vi "Write command to PG.vi"(8 "error in (no error)":errorcluster, 10 "Write Buffer":string, 11 "VISA resource name":refnum<visa-resource-name>) -> (0 "error out":errorcluster, 2 "Read Buffer":string, 3 "VISA resource name out":refnum<visa-resource-name>)   [LabVIEW 2018]
uses:
  <vilib>/Utility/error.llb/DialogType.ctl
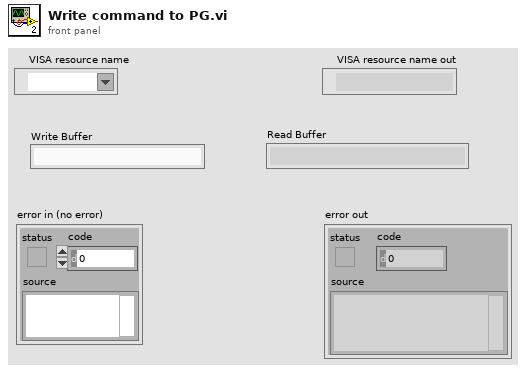
[diagram p1: front panel]
types:
  T1 = typedef "DialogType.ctl" = u16
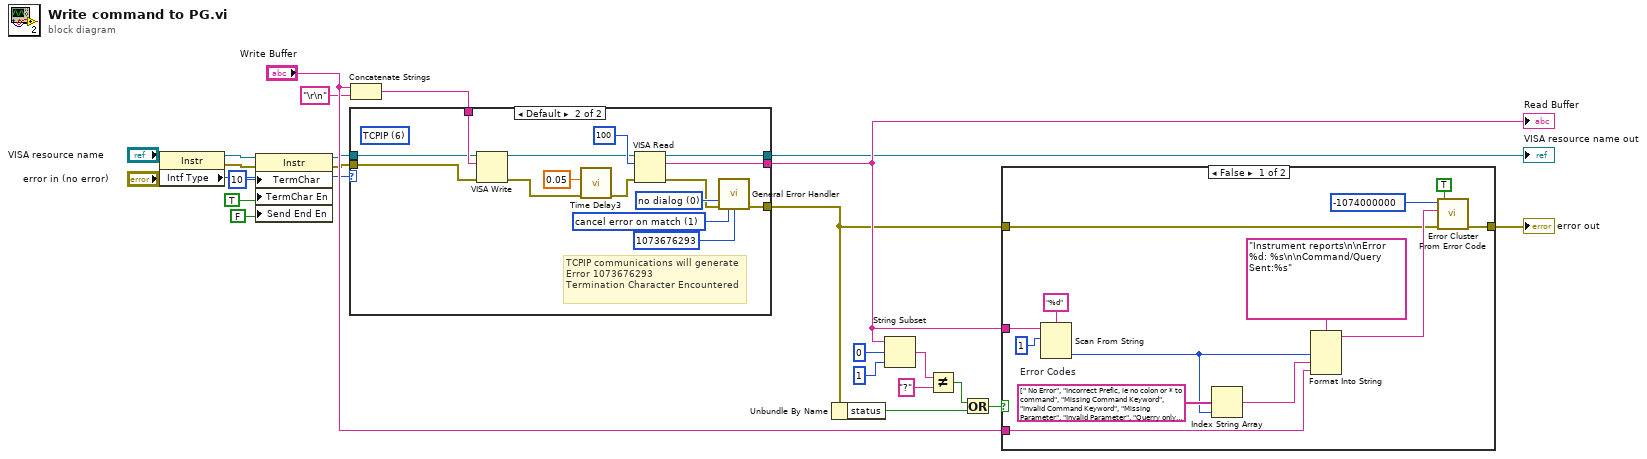
[diagram p0: block diagram]
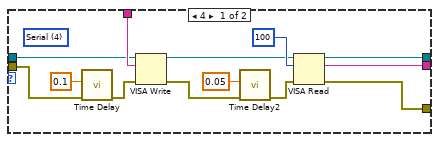
[diagram p2: hidden frame]
diagram:
  n1 = property class="Instr"(reference="VISA resource name", error in="error in (no error)") -> (reference out=w6:refnum<visa-resource-name>, error out=w7:errorcluster, "Intf Type"=w9:u16)
  n2 = property class="Instr"(reference=w6, error in=w7, "TermChar"=u8 10 ("Message Based Settings:Termination Character"), "TermChar En"=TRUE ("Message Based Settings:Termination Character Enable"), "Send End En"=FALSE ("Message Based Settings:Send End Enable")) -> (reference out=w5:refnum<visa-resource-name>, error out=w4:errorcluster)
  n3 = Concatenate Strings("Write Buffer", "\r\n" ("string")) -> (w24:string)
  n4 = case shown="Default" w9 {
    tunnel: w24 -> [w37 w52]
    tunnel: [w35 w50] -> w19
    tunnel: [w34 w49] -> w14
    tunnel: [w33 w38] -> w8
    tunnel: w5 -> [w29 w46]
    tunnel: w4 -> [w28 w43]
    frame 4 {
      (unwired) u16 4 items=["GPIB"=1, "VXI"=2, "GPIB-VXI"=3, "Serial"=4, "PXI"=5, "TCPIP"=6, "USB"=7, "FireWire"=9] ("Interface Information:Interface Type")
      n5 = call "Time Delay"("error in (no error)"=w28, "Delay Time (s)"=0.1) -> ("error out"=w30:errorcluster)  [unwired: 9 out]
      n6 = VISA Write(VISA resource name=w29, write buffer=w37, error in (no error)=w30) -> (VISA resource name out=w27:refnum<visa-resource-name>, error out=w31:errorcluster)  [unwired: 1 out]
      n7 = call "Time Delay2"("error in (no error)"=w31, "Delay Time (s)"=0.05) -> ("error out"=w32:errorcluster)  [unwired: 9 out]
      n8 = VISA Read(VISA resource name=w27, byte count=u32 100, error in (no error)=w32) -> (VISA resource name out=w34:refnum<visa-resource-name>, read buffer=w35:string, error out=w33:errorcluster)  [unwired: 1 out]
    }
    frame Default {
      w42 = T1 0 items=["no dialog", "OK message", "continue or stop message", "OK message + warnings", "continue/stop + warnings"] ("type of dialog (OK msg:1)")
      (unwired) u16 6 items=["GPIB"=1, "VXI"=2, "GPIB-VXI"=3, "Serial"=4, "PXI"=5, "TCPIP"=6, "USB"=7, "FireWire"=9] ("Interface Information:Interface Type")
      w40 = 1 items=["no exception", "cancel error on match", "set error on match"] ("[exception action] (none:0)")
      # "TCPIP communications will generate\nError 1073676293\nTermination Character Encountered"
      n9 = VISA Write(VISA resource name=w46, write buffer=w52, error in (no error)=w43) -> (VISA resource name out=w45:refnum<visa-resource-name>, error out=w47:errorcluster)  [unwired: 1 out]
      n10 = call "Time Delay3"("error in (no error)"=w47, "Delay Time (s)"=0.05) -> ("error out"=w48:errorcluster)  [unwired: 9 out]
      n11 = VISA Read(VISA resource name=w45, byte count=u32 100, error in (no error)=w48) -> (VISA resource name out=w49:refnum<visa-resource-name>, read buffer=w50:string, error out=w39:errorcluster)  [unwired: 1 out]
      n12 = call <vilib>:"General Error Handler.vi"("type of dialog (OK msg:1)"=w42, "error in (no error)"=w39, "[exception action] (none:0)"=w40, "[exception code]"=1073676293) -> ("error out"=w38:errorcluster)  [unwired: 2 in, 9 out]
    }
  }
  "Read Buffer" <- w19
  "VISA resource name out" <- w14
  n13 = Unbundle By Name(w8) -> ("status"=w15:bool)
  n14 = String Subset(string=w19, offset (0)=0, length (rest)=1 ("length (rest)")) -> (substring=w16:string)
  n15 = Not Equal?(x=w16, y="?" ("x")) -> (x != y?=w18:bool)
  n16 = Or(x=w18, y=w15) -> (x .or. y?=w23:bool)
  n17 = case shown="False" w23 {
    tunnel: w19 -> [w64 _]
    tunnel: [w55 w66] -> w22
    tunnel: w8 -> [w53 w66]
    tunnel: "Write Buffer" -> [w59 _]
    frame False {
      w62 = string[] [" No Error", "Incorrect Prefic, ie no colon or * to command", "Missing Command Keyword", "Invalid Command Keyword", "Missing Parameter", "Invalid Parameter", "Querry only, command needs a question mark", "Invalid Query, command does not have a query form"]  # Error Codes
      n18 = Scan From String(format string="%d" ("Format String"), input string=w64, initial scan location=u32 1) -> (output 1=w61:i32)  [unwired: 1 in, 4 out]
      n19 = Index String Array(1:w61, 2:w62) -> (0:w60:string)  [unwired: 1 out]
      n20 = Format Into String(format string="Instrument reports\n\nError %d: %s\n\nCommand/Query Sent:%s" ("Source"), w61, w60, w59) -> (resulting string=w54:string)  [unwired: 2 in, 1 out]
      n21 = call <vilib>:"Error Cluster From Error Code.vi"("show call chain? (False)"=TRUE, "error in (no error)"=w53, "error message (\"\")"=w54, "error code (0)"=-1074000000 ("Code")) -> ("error out"=w55:errorcluster)  [unwired: 5 out]
    }
    frame True {
    }
  }
  "error out" <- w22
